vi "Dashboard Main.vi"() -> ()   [LabVIEW 2018]
uses:
  2019_Trobots_5013_Robot/Arm/Arm Positions.ctl
  <vilib>/Utility/miscctls.llb/LVRowAndColumnTypeDef.ctl
  <vilib>/event_ctls.llb/eventvkey.ctl
  <vilib>/Rock Robotics/Network Tables/NT Read Numeric Array.vi
  <vilib>/Rock Robotics/WPI/Dashboard/WPI_DashboardLogging Global.vi
panel:
  in  "Camera Settings Right":T1={"Frame Rate"=30, "Compression"=30, "Size"=1, "DB Camera Config"=FALSE} {"Frame Rate" scale=1.0..30.0; "Compression" scale=100.0..-1.0; "Size" items=["640x480", "320x240", "160x120"]}
  in  "Camera Name Right":string(combo)="No Camera Selection"
  out "Camera Perf":string
  in  "Camera Settings":T1={"Frame Rate"=30, "Compression"=30, "Size"=1, "DB Camera Config"=FALSE} {"Frame Rate" scale=1.0..30.0; "Compression" scale=100.0..-1.0; "Size" items=["640x480", "320x240", "160x120"]}
  in  "TCP":refnum<k5>
  in  "Rec Mode":enum32{"Stop", "Record", "Playback"}(radio)
  out "Robot IP":string
  out "Image Message":string="Timeout in Camera Communications"
  in  "Dashboard Tab":T2(tab)=enum."Custom"
  in  "Select Auto":string(combo)="Select Autonomous ..."
  out "NT Connection":bool
  out "MotorChart R":cluster{"Numeric":dbl, "Numeric":dbl}(graph)
  out "MotorChart L":cluster{"Numeric":dbl, "Numeric":dbl}(graph)
  out "MotorSliders R":cluster{"MotorSlide1":dbl, "MotorSlide2":dbl} {"MotorSlide2" scale=-1.0..1.0 scale format="%#_2e"; "MotorSlide1" scale=-1.0..1.0 scale format="%#_2e"}
  out "MotorSliders L":cluster{"MotorSlide1":dbl, "MotorSlide2":dbl} {"MotorSlide2" scale=-1.0..1.0 scale format="%#_2e"; "MotorSlide1" scale=-1.0..1.0 scale format="%#_2e"}
  out "JS1 Z":dbl(slide) scale=-1.0..1.0 scale format="%#_2e"
  out "JS1 Graph":cluster{"X":dbl, "Y":dbl}[](graph)
  out "JS1 Buttons":T3
  out "JS2 Z":dbl(slide) scale=-1.0..1.0 scale format="%#_2e"
  out "JS2 Graph":cluster{"X":dbl, "Y":dbl}[](graph)
  out "JS2 Buttons":T3
  out "Mode":T4(ring)=enum."Auto Disabled"
  out "Right Camera Perf":cluster{"Bandwidth (Mbps)":dbl, "FPS":dbl}
  out "Camera Image Right":T5(plugin-control)
  in  "DB/String 9":string
  in  "DB/String 8":string
  in  "DB/String 7":string
  in  "DB/String 6":string
  in  "DB/String 5":string
  in  "DB/String 4":string
  in  "DB/String 3":string
  in  "DB/String 2":string
  in  "DB/String 1":string
  in  "DB/String 0":string
  in  "DB/Slider 0":dbl(slide) scale=0.0..5.0
  in  "DB/Slider 1":dbl(slide) scale=0.0..5.0
  in  "DB/Slider 2":dbl(slide) scale=0.0..5.0
  in  "DB/Slider 3":dbl(slide) scale=0.0..5.0
  out "DB/LED 3":bool
  out "DB/LED 2":bool
  out "DB/LED 1":bool
  out "DB/LED 0":bool
  in  "DB/Button 3":bool
  in  "DB/Button 2":bool
  in  "DB/Button 1":bool
  in  "DB/Button 0":bool caption="New Name"
  in  "Array":bool[](array[boolean])
  in  "Set":bool
  in  "Elbow Angle":dbl
  in  "Shoulder Angle":dbl
  in  "Wrist Angle":dbl
  in  "Turret Angle":dbl
  in  "Arm Positions":T6
  out "Elbow":dbl format="%#.1f"
  out "Turret":dbl format="%#.1f"
  out "Shoulder":dbl format="%#.1f"
  out "Wrist":dbl format="%#.1f"
  out "Gyro":dbl(knob) scale=-180.0..180.0
  in  "Test Slider":dbl(slide) scale=0.0..100.0 scale format="%#_3g"
  in  "On/Off":bool caption="Solenoid"
  in  "Test Name":u16(ring) items=["Select the test to run..."]
  in  "Test Tree":string(tree)
  in  "Motor":cluster{"Value":dbl, "Enable":bool} {"Value" scale=-1.0..1.0 scale format="%#_3g"}
  out "Progress":T7 {"Test Progress" scale=0.0..100.0}
  in  "Rev/Fwd":cluster{"Forward":bool, "Reverse":bool}
  in  "Test Ring":u16(ring) items=["Monochrome", "Color"]
  out "Cmd Status":string
  in  "Execute Command":bool
  in  "Command Params":string[][](table)
  in  "Command Selection":i32(listbox)
  in  "CheckList":i32(listbox)
  out "Tree":string(tree)
  out "Camera Image":T5(plugin-control)
  out "Background":bool
  in  "Camera Name":string(combo)="No Camera Selection"
  # "HW"
  # "HW"
  # "Joysticks"
  # "Drive Motors"
  # "Front"
  # "Right"
  # "Left"
  # "Back"
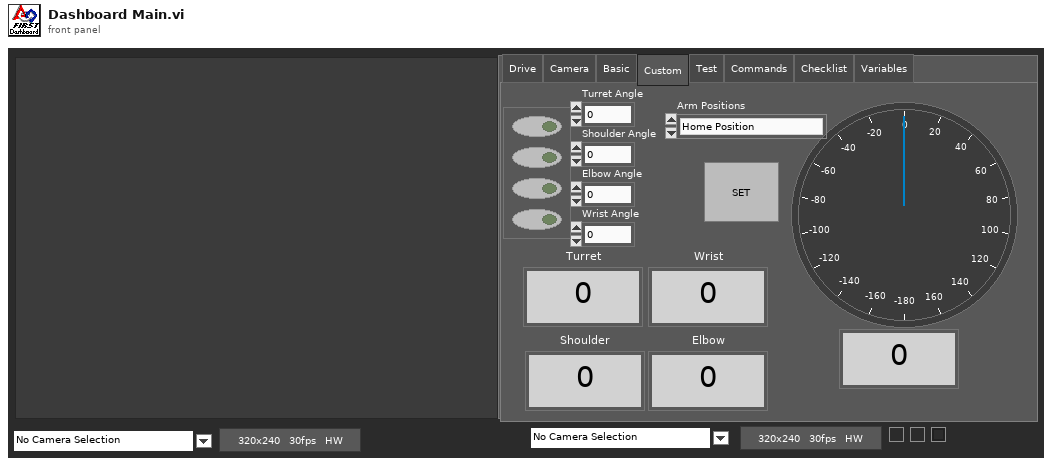
[diagram p1: front panel]
types:
  T1 = cluster{"Frame Rate":i32, "Compression":i32, "Size":u16, "DB Camera Config":bool}
  T2 = enum32{"Drive", "Camera", "Basic", "Custom", "Test", "Commands", "Checklist", "Variables"}
  T3 = cluster{bool, bool, bool, bool, bool, bool, bool, bool, bool, bool, bool, bool}
  T4 = enum8{"Tele-Op Disabled", "Tele-Op Enabled", "Auto Disabled", "Auto Enabled", "Test Disabled", "Test Enabled", "Disconnected", "No Code", "E-Stop"}
  T5 = typedef "IMAQ Image.ctl" = refnum<image>
  T6 = typedef "Arm Positions.ctl" = enum16{"Home Position", "Safe Position", "Hatch - Ground", "Hatch - Low", "Hatch - Middle", "Hatch - High", "Hatch - High 2", "Cargo - Low", "Cargo - Middle", "Cargo - High", "Cargo - Loading Station", "Hatch - Loading Station", "Cargo - Ground", "Turret - Left", "Turret - Front", "Turret - Right", "Turret - Back", "Climbing - Forward", "Hatch - Middle2"}
  T7 = cluster{"Test Progress":u8, "Test Progress Text":string}
  T8 = cluster{"Save Path":path, "Interval (s)":dbl, "Keep":i32}
  T9 = typedef "Image Type" = u32
  T10 = cluster{"IDs":cluster{"RPC field ID":u16, "Unique ID":u16}, "String":string}
  T11 = cluster{"Error Strings":string, "Disable Counts":cluster{u16, u16}, "Rail Faults":cluster{u16, u16, u16}, "Robot IP":string, "DB Mode":u8, "Event Info":cluster{"Name":string, "Type":u8, "Number":u16, "Replay":u8}}
  T12 = cluster{"Storage":cluster{"Disk Free":u64, "RAM Block":u32, "RAM free":u32}, "CPU Utilization":cluster{"CPU % ISR":sgl, "CPU % Time Crit":sgl, "CPU % Timed Str":sgl, "CPU % High":sgl, "CPU % Above":sgl, "CPU % Normal":sgl, "CPU % Low":sgl}, "CAN":cluster{"% Bus Utilization":sgl, "Bus Off Cnt":u32, "TX_FIFO Full Cnt":u32, "Receive Error Cnt":u8, "Transmit Error Cnt":u8}, "HID":cluster{"HID Outputs":u32, "Rumble Low":u16, "Rumble High":u16}[]}
  T13 = cluster{"Status bits":cluster{"Test Mode":bool, "Autonomous":bool, "Enabled":bool, "Code Start":bool, "Brownout":bool, "Reserved 2":bool, "Reserved 3":bool, "E-Stop":bool}, "Code Trace":cluster{"Disabled":bool, "TeleOp":bool, "Auto":bool, "Test":bool}, "Controller Type":enum16{"unknown", "cRIO", "roboRio"}, "Code?":enum16{"unknown", "noCode", "code"}, "Battery V":dbl}
  T14 = cluster{"Control Bits":cluster{"TestMode":bool, "Autonomous":bool, "Enabled":bool, "FMS Present":bool, bool, bool, bool, "E-Stop":bool}, "Team Station ":u8, "Countdown":sgl, "Joystick Values":cluster{"Axes":dbl[], "Buttons":bool[], "POVs":i16[]}[]}
  T15 = cluster{"Axes":dbl[], "Buttons":bool[], "POVs":i16[]}[]
  T16 = cluster{"Axes":dbl[], "Buttons":bool[], "POVs":i16[]}
  T17 = cluster{"Buttons[0]":bool, "Buttons[1]":bool, "Buttons[2]":bool, "Buttons[3]":bool, "Buttons[4]":bool, "Buttons[5]":bool, "Buttons[6]":bool, "Buttons[7]":bool, "Buttons[8]":bool, "Buttons[9]":bool, "Buttons[10]":bool, "Buttons[11]":bool}
  T18 = cluster{"Camera Image":refnum<vi>, "Dashboard Tab":refnum<vi>, "Background":refnum<vi>, "Rec Mode":refnum<vi>, "Test Slider":refnum<vi>, "On/Off ":refnum<vi>, "Test Ring":refnum<vi>, "Rev/Fwd":refnum<vi>, "Test Name":refnum<vi>, "Motor":refnum<vi>, "Progress":refnum<vi>, "CheckList":refnum<vi>, "Tree":refnum<vi>, "Test Tree":refnum<vi>, "Command Params":refnum<vi>, "Command Selection":refnum<vi>, "Execute Command":refnum<vi>, "Cmd Status":refnum<vi>, "Camera Settings":refnum<vi>, "Camera Name":refnum<vi>, "Camera Perf":refnum<vi>, "Camera Settings Right":refnum<vi>, "Camera Name Right":refnum<vi>, "Camera Image Right":refnum<vi>}
  T19 = cluster{"Global Rectangle":i32[], "Contours":cluster{"Contour Type":u32, "ROI Type":u32, "Points":i32[]}[]}
  T20 = cluster{"Camera Name":string, string, "Saved DB Images Info":cluster{"Save Path":path, "Interval (s)":dbl, "Keep":i32}}
  T21 = cluster{"Camera Name Right":string, string, "Saved DB Images Info":cluster{"Save Path":path, "Interval (s)":dbl, "Keep":i32}}
  T22 = cluster{"Operation":enum16{"Update", "Clear"}, "Color Box":u32}[]
  T23 = typedef "eventvkey.ctl" = enum16{"ASCII", "Enter", "Return", "Shift", "Ctrl", "Alt", "Cmd", "Opt", "Caps", "NumLock", "Clear", "Break", "Up", "Down", "Left", "Right", "Insert", "Delete", "Home", "End", "PageUp", "PageDown", "Escape", "Help", "Pause", "ScrollLock", "F1", "F2", "F3", "F4", "F5", "F6", "F7", "F8", "F9", "F10", "F11", "F12", "F13", "F14", "F15", "F16", "F17", "F18", "F19", "F20", "F21", "F22", "F23", "F24", "Play", "VolumeUp", "VolumeDown", "Mute", "Two Byte Char"}
  T24 = cluster{"Image Size":bool, "Image Type":bool, "Pixel Value":bool, "ROI Information":bool, "Zoom Factor":bool}
  T25 = cluster{"Operation":enum16{"Update", "Clear"}, "Color Box":u32}
  T26 = typedef "LVRowAndColumnTypeDef.ctl" = cluster{"Row":i32, "Column":i32}
  T27 = cluster{"Shift":bool, "Ctrl":bool, "Alt":bool, "Cmd":bool, "Opt":bool}
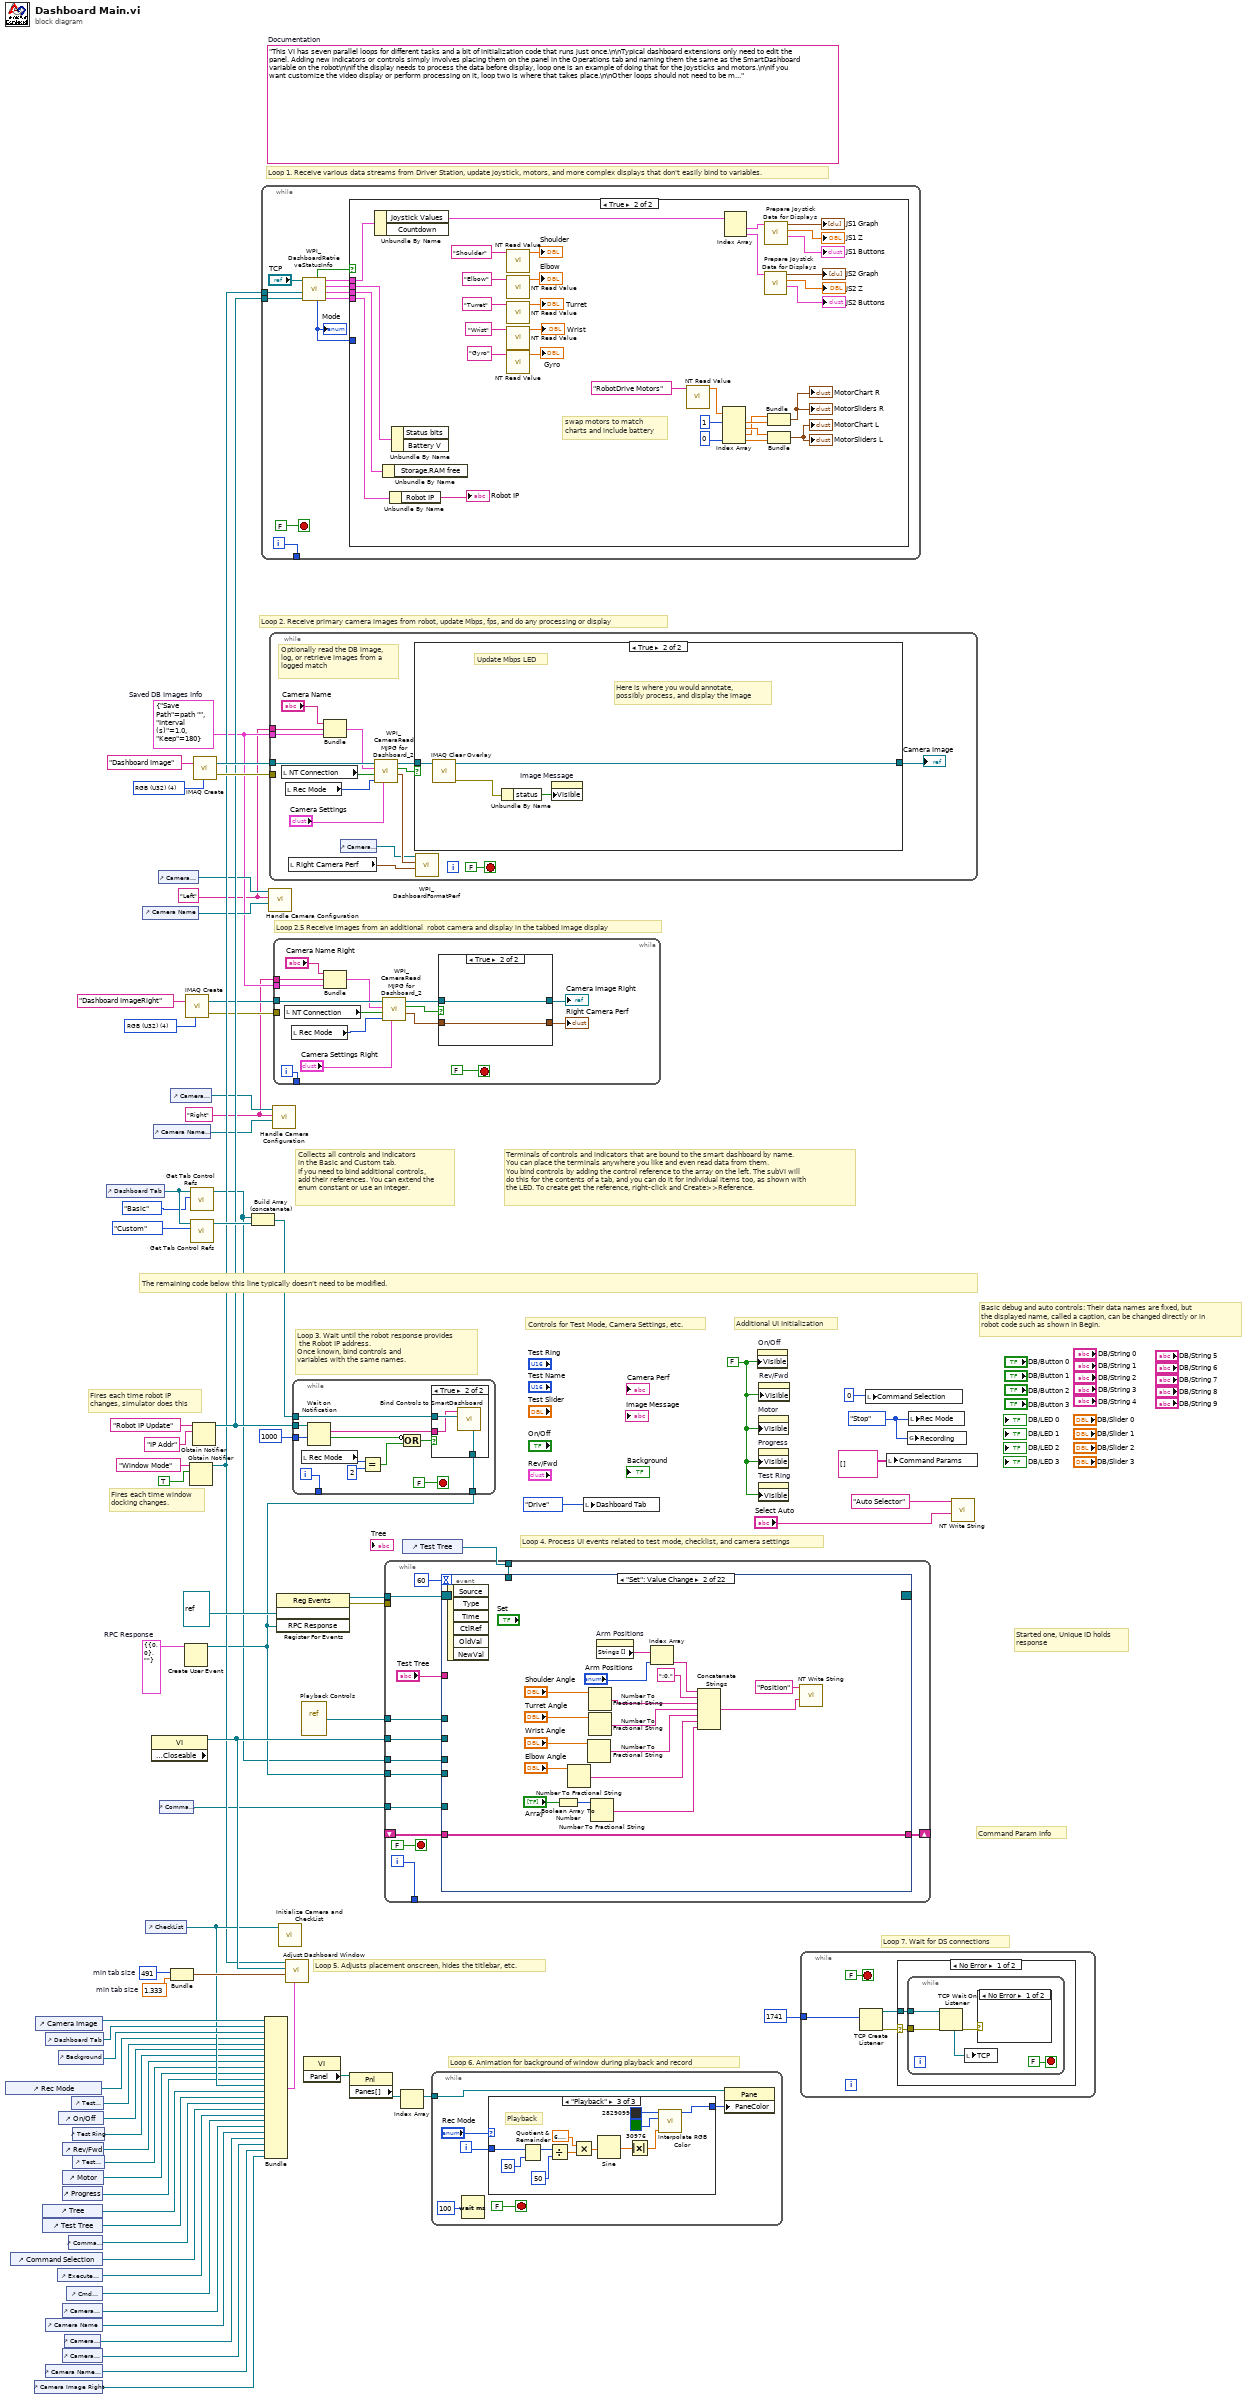
[diagram p0: block diagram]
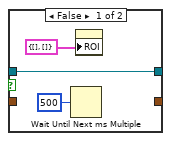
[diagram p2: hidden frame]
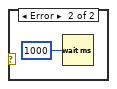
[diagram p3: hidden frame]
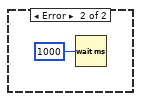
[diagram p4: hidden frame]
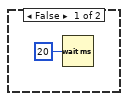
[diagram p5: hidden frame]
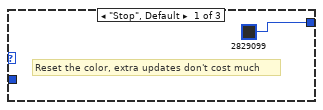
[diagram p6: hidden frame]
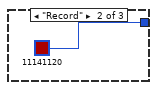
[diagram p7: hidden frame]
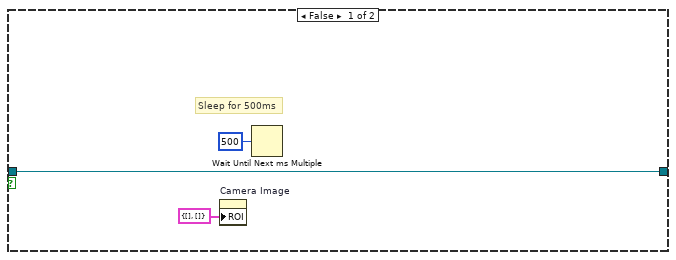
[diagram p9: hidden frame]
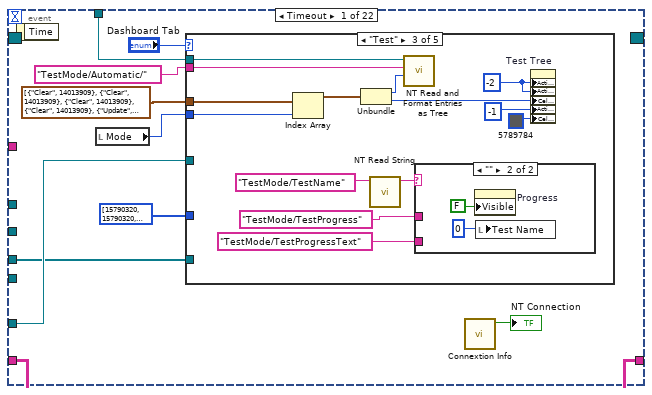
[diagram p10: hidden frame]
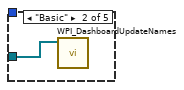
[diagram p12: hidden frame]
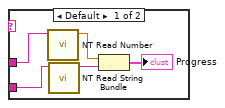
[diagram p13: hidden frame]
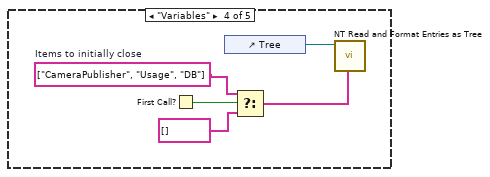
[diagram p14: hidden frame]
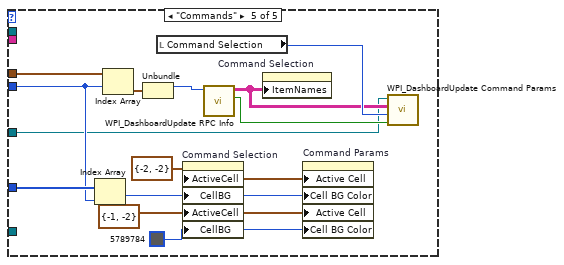
[diagram p15: hidden frame]
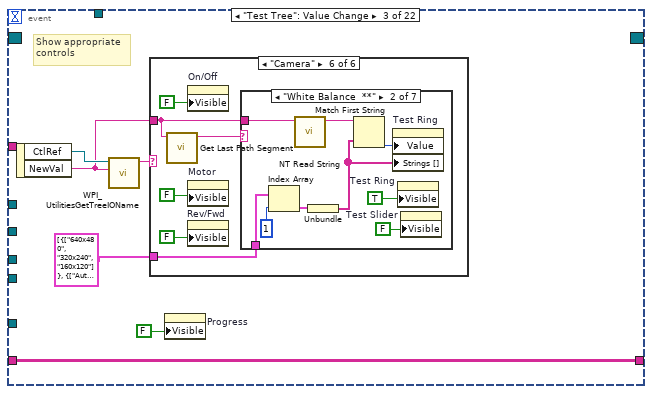
[diagram p16: hidden frame]
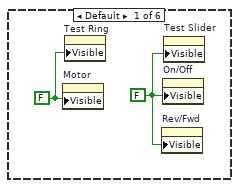
[diagram p17: hidden frame]
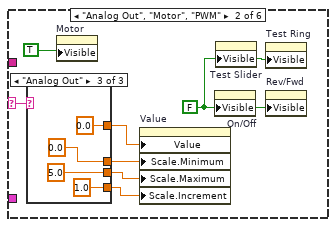
[diagram p18: hidden frame]
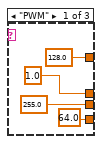
[diagram p19: hidden frame]
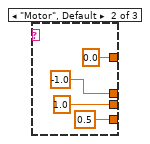
[diagram p20: hidden frame]
diagram:
  w3 = T8 {"Save Path"=path "", "Interval (s)"=1.0, "Keep"=180}  # Saved DB Images Info
  w2 = "Right"
  w1 = "Left"
  w13 = T9 4 items=["Grayscale (U8)", "Grayscale (I16)", "Grayscale (SGL)", "Complex (CSG)", "RGB (U32)", "HSL (U32)", "RGB (U64)"] ("Image Type")
  w29 = T10 {"IDs"={"RPC field ID"=0, "Unique ID"=0}, "String"=""}  # RPC Response
  w52 = 491  # min tab size
  w51 = 1.333  # min tab size
  w59 = enum32{"Stop", "Record", "Playback"}."Stop" ("Rec Mode")
  w36 = FALSE ("Visible")
  (unwired) "This VI has seven parallel loops for different tasks and a bit of initialization code that runs just once.\n\nTypical dashboard extensions only need to edit the panel. Adding new indicators or controls simply involves placing them on the panel in the Operations tab and naming them the same as the SmartDashboard variable on the robot\n\nIf the display needs to process the data before display, loop one is an example of doing that for the joysticks and motors.\n\nIf you want customize the video display or perform processing on it, loop two is where that takes place.\n\nOther loops should not need to be modified. They are pretty standard, and document the task they perform."  # Documentation
  w76 = T9 4 items=["Grayscale (U8)", "Grayscale (I16)", "Grayscale (SGL)", "Complex (CSG)", "RGB (U32)", "HSL (U32)", "RGB (U64)"] ("Image Type")
  # "Loop 2.5 Receive images from an additional  robot camera and display in the tabbed image display"
  # "Command Param Info"
  # "Started one, Unique ID holds\nresponse"
  # "Loop 7. Wait for DS connections"
  # "Basic debug and auto controls: Their data names are fixed, but\nthe displayed name, called a caption, can be changed directly or in\nrobot code such as shown in Begin."
  # "Controls for Test Mode, Camera Settings, etc."
  # "Additional UI Initialization"
  # "Loop 6. Animation for background of window during playback and record"
  # "Fires each time robot IP\nchanges, simulator does this"
  # "Fires each time window\ndocking changes."
  # "Collects all controls and indicators\nin the Basic and Custom tab.\nIf you need to bind additional controls,\nadd their references. You can extend the\nenum constant or use an integer."
  # "The remaining code below this line typically doesn't need to be modified."
  # "Loop 4. Process UI events related to test mode, checklist, and camera settings"
  # "Terminals of controls and indicators that are bound to the smart dashboard by name.\nYou can place the terminals anywhere you like and even read data from them.\nYou bind controls by adding the control reference to the array on the left. The subVI will\ndo this for the contents of a tab, and you can do it for individual items too, as shown with\nthe LED. To create get the reference, right-click and Create>>Reference."
  # "Loop 3. Wait until the robot response provides\n the Robot IP address.\nOnce known, bind controls and\nvariables with the same names."
  # "Loop 5. Adjusts placement onscreen, hides the titlebar, etc."
  # "Loop 1. Receive various data streams from Driver Station, update joystick, motors, and more complex displays that don't easily bind to variables."
  # "Loop 2. Receive primary camera images from robot, update Mbps, fps, and do any processing or display"
  n1 = control-ref of="Rec Mode"() -> (w42:refnum<vi>)
  n2 = control-ref of="Command Selection"() -> (w28:refnum<vi>)
  n3 = control-ref of="Camera Image Right"() -> (w6:refnum<vi>)
  n4 = control-ref of="Camera Image"() -> (w54:refnum<vi>)
  n5 = control-ref of="Tree"() -> (w46:refnum<vi>)
  n6 = control-ref of="Test Tree"() -> (w45:refnum<vi>)
  n7 = control-ref of="Dashboard Tab"() -> (w53:refnum<vi>)
  n8 = control-ref of="Camera Name"() -> (w19:refnum<vi>)
  n9 = control-ref of="Camera Name Right"() -> (w7:refnum<vi>)
  n10 = control-ref of="Execute Command"() -> (w30:refnum<vi>)
  n11 = control-ref of="Background"() -> (w49:refnum<vi>)
  n12 = control-ref of="On/Off"() -> (w40:refnum<vi>)
  n13 = control-ref of="Progress"() -> (w37:refnum<vi>)
  n14 = control-ref of="Camera Settings"() -> (w20:refnum<vi>)
  n15 = control-ref of="Camera Settings Right"() -> (w8:refnum<vi>)
  n16 = control-ref of="Rev/Fwd"() -> (w38:refnum<vi>)
  n17 = control-ref of="Motor"() -> (w43:refnum<vi>)
  n18 = control-ref of="Camera Perf"() -> (w18:refnum<vi>)
  n19 = control-ref of="Cmd Status"() -> (w24:refnum<vi>)
  n20 = control-ref of="Command Params"() -> (w31:refnum<vi>)
  n21 = control-ref of="Test Slider"() -> (w41:refnum<vi>)
  n22 = control-ref of="Test Ring"() -> (w39:refnum<vi>)
  n23 = control-ref of="Test Name"() -> (w44:refnum<vi>)
  n24 = control-ref of="Dashboard Tab"() -> (w57:refnum<vi>)
  n25 = control-ref of="Camera Name"() -> (w21:refnum<vi>)
  n26 = control-ref of="CheckList"() -> (w47:refnum<vi>)
  n27 = property class="VI" props=["Front Panel.Closeable"]() -> (reference out=w58:refnum<vi>)  [unwired: 2 in, 2 out]
  n28 = control-ref of="Camera Name Right"() -> (w9:refnum<vi>)
  n29 = control-ref of="Camera Settings"() -> (w22:refnum<vi>)
  n30 = control-ref of="Command Params"() -> (w23:refnum<vi>)
  n31 = control-ref of="Camera Settings Right"() -> (w10:refnum<vi>)
  n32 = Bundle("min tab size"=w52, "min tab size"=w51) -> (w50:cluster{"min tab size":i32, "min tab size":dbl})  [unwired: 1 in]
  n33 = Create User Event(user event datatype=w29) -> (user event=w25:refnum<user-event>)  [unwired: 1 in, 1 out]
  n34 = call "IMAQ Create"("Image Name"="Dashboard ImageRight", "Image Type"=w13) -> ("New Image"=w12:T5, "error out"=w11:errorcluster)  [unwired: 2 in, 1 out]
  n35 = Obtain Notifier(name (unnamed)="Window Mode", notification data type=TRUE) -> (notifier out=w34:refnum<notifier>)  [unwired: 2 in, 2 out]
  n36 = call <vilib>:"Get Tab Control Refs.vi"("Page Index"=T2."Basic" ("Dashboard Tab"), "TabControl in"=w57) -> ("ControlsOnPage"=w17:refnum<vi>[])  [unwired: 9 in]
  n37 = call <vilib>:"Get Tab Control Refs.vi"("Page Index"=T2."Custom" ("Dashboard Tab"), "TabControl in"=w57) -> ("ControlsOnPage"=w56:refnum<vi>[])  [unwired: 9 in]
  n38 = Obtain Notifier(name (unnamed)="Robot IP Update", notification data type="IP Addr" ("name (unnamed)")) -> (notifier out=w35:refnum<notifier>)  [unwired: 2 in, 2 out]
  n39 = call "IMAQ Create"("Image Name"="Dashboard Image", "Image Type"=w76) -> ("New Image"=w74:T5, "error out"=w73:errorcluster)  [unwired: 2 in, 1 out]
  n40 = Build Array (concatenate)(w17, w56) -> (w55:refnum<vi>[])
  n41 = while {
    tunnel: [w86] -> _
    tunnel: w35 -> [w80]
    tunnel: w34 -> [w77]
    i -> [w86]
    stop <- FALSE stop-if-true
    n42 = call <vilib>:"WPI_DashboardRetrieveStatusInfo.vi"("Binding Refnum"=w80, "Window Mode Notifier"=w77, "TCP Cnx"="TCP") -> ("Power and Errors"=w81:T11, "Robot Metrics"=w84:T12, "Status Info"=w85:T13, "Control Info"=w82:T14, "Robot Mode"=w79:T4, "Process?"=w83:bool)  [unwired: 3 in]
    "Mode" <- w79
    n43 = case shown="True" w83 {
      tunnel: w85 -> [_ w122]
      tunnel: w84 -> [_ w121]
      tunnel: w82 -> [_ w120]
      tunnel: w81 -> [_ w119]
      tunnel: w79 -> [_ _]
      frame False {
        n44 = Wait (ms)(milliseconds to wait=u32 20) -> ()  [unwired: 1 out]
      }
      frame True {
        # "swap motors to match\ncharts and include battery"
        n45 = Unbundle By Name(w120) -> ("Joystick Values"=w110:T15)  [unwired: 1 out]
        n46 = Unbundle By Name(w121) -> ()  [unwired: 1 out]
        n47 = Unbundle By Name(w119) -> ("Robot IP"=→"Robot IP":string)
        n48 = Unbundle By Name(w122) -> ()  [unwired: 2 out]
        n49 = call-poly <vilib>:"NT Read Value.vi"("Name"="Shoulder") -> ("Numeric"=→"Shoulder":dbl)  [unwired: 9 in, 1 out]
        n50 = call-poly <vilib>:"NT Read Value.vi"("Name"="Elbow") -> ("Numeric"=→"Elbow":dbl)  [unwired: 9 in, 1 out]
        n51 = call-poly <vilib>:"NT Read Value.vi"("Name"="Turret") -> ("Numeric"=→"Turret":dbl)  [unwired: 9 in, 1 out]
        n52 = call-poly <vilib>:"NT Read Value.vi"("Name"="Wrist") -> ("Numeric"=→"Wrist":dbl)  [unwired: 9 in, 1 out]
        n53 = call-poly <vilib>:"NT Read Value.vi"("Name"="Gyro") -> ("Numeric"=→"Gyro":dbl)  [unwired: 9 in, 1 out]
        n54 = call-poly <vilib>:"NT Read Value.vi"("Name"="RobotDrive Motors") -> ("Numeric Array"=w100:dbl[])  [unwired: 9 in, 1 out]
        n55 = Index Array(array=w100, index #1=1, index #4=0) -> (element #1=w114:dbl, element #2=w115:dbl, element #3=w113:dbl, element #4=w118:dbl)  [unwired: 2 in]
        n56 = Index Array(array=w110) -> (element #1=w109:T16, element #2=w105:T16)  [unwired: 2 in]
        n57 = call "Prepare Joystick Data for Displays.vi"("Joystick Values"=w105) -> ("Buttons"=→"JS2 Buttons":T17, "Z Axis"=→"JS2 Z":dbl, "Cartesian Data"=→"JS2 Graph":cluster{"X axis":dbl, "X axis":dbl}[])  [unwired: 8 in]
        n58 = call "Prepare Joystick Data for Displays.vi"("Joystick Values"=w109) -> ("Buttons"=→"JS1 Buttons":T17, "Z Axis"=→"JS1 Z":dbl, "Cartesian Data"=→"JS1 Graph":cluster{"X axis":dbl, "X axis":dbl}[])  [unwired: 8 in]
        n59 = Bundle("Numeric"=w113, "Numeric"=w114) -> (→"MotorChart R" →"MotorSliders R":cluster{"Numeric":dbl, "Numeric":dbl})  [unwired: 1 in]
        n60 = Bundle("Numeric"=w115, "Numeric"=w118) -> (→"MotorChart L" →"MotorSliders L":cluster{"Numeric":dbl, "Numeric":dbl})  [unwired: 1 in]
      }
    }
  }
  n61 = Bundle("Camera Image"=w54, "Dashboard Tab"=w53, "Background"=w49, "Rec Mode"=w42, "Test Slider"=w41, "On/Off"=w40, "Test Ring"=w39, "Rev/Fwd"=w38, "Test Name"=w44, "Motor"=w43, "Progress"=w37, "CheckList"=w47, "Tree"=w46, "Test Tree"=w45, "Command Params"=w31, "Command Selection"=w28, "Execute Command"=w30, "Cmd Status"=w24, "Camera Settings"=w20, "Camera Name"=w19, "Camera Perf"=w18, "Camera Settings Right"=w8, "Camera Name Right"=w7, "Camera Image Right"=w6) -> (w48:T18)  [unwired: 1 in]
  n62 = call "Handle Camera Configuration.vi"("CameraNameRef"=w21, "Display Name"=w1, "ClusterRef"=w22) -> ()  [unwired: 9 in]
  n63 = while {
    tunnel: w74 -> [w136]
    tunnel: w73 -> [_]
    tunnel: w3 -> [w129]
    tunnel: w1 -> [w126]
    stop <- FALSE stop-if-true
    # "Optionally read the DB image,\nlog, or retrieve images from a\nlogged match"
    n64 = local read "NT Connection"() -> (w130:bool)
    n65 = local read "Rec Mode"() -> (w133:enum32{"Stop", "Record", "Playback"})
    n66 = local read "Right Camera Perf"() -> (w124:cluster{"Bandwidth (Mbps)":dbl, "FPS":dbl})
    n67 = Bundle("Camera Name"="Camera Name", w126, "Saved DB Images Info"=w129) -> (w128:T20)  [unwired: 1 in]
    n68 = control-ref of="Camera Perf"() -> (w123:refnum<vi>)
    n69 = call <vilib>:"WPI_CameraRead MJPG for Dashboard_2.vi"("Camera Settings"="Camera Settings", "Rec Mode"=w133, "NT Connection"=w130, "Capture Info"=w128, "Image in"=w136) -> ("perf info"=w125:cluster{"Bandwidth (Mbps)":dbl, "fps":dbl}, "Active"=w134:bool, "Image\\ out"=w135:T5)  [unwired: 4 in]
    n70 = case shown="True" w134 {
      tunnel: w135 -> [w139 w142]
      tunnel: [w139 w141] -> w131
      frame False {
        # "Sleep for 500ms"
        n71 = property on="Camera Image" class="ImageControl"("ROI"=T19 {"Global Rectangle"=[], "Contours"=[]}) -> ()  [unwired: 2 in, 2 out]
        n72 = Wait Until Next ms Multiple(millisecond multiple=u32 500) -> ()  [unwired: 1 out]
      }
      frame True {
        # "Here is where you would annotate,\npossibly process, and display the image"
        # "Update Mbps LED"
        n73 = call "IMAQ Clear Overlay"("Image"=w142) -> ("error out"=w143:errorcluster, "Image Out"=w141:T5)  [unwired: 2 in, 7 out]
        n74 = Unbundle By Name(w143) -> ("status"=w144:bool)
        n75 = property on="Image Message" class="Str"("Visible"=w144) -> ()  [unwired: 2 in, 2 out]
      }
    }
    "Camera Image" <- w131
    n76 = call <vilib>:"WPI_DashboardFormatPerf.vi"("Right Camera Perf"=w124, "Performance"=w125, "String in"=w123) -> ()  [unwired: 9 in]
  }
  n77 = call "Handle Camera Configuration.vi"("CameraNameRef"=w9, "Display Name"=w2, "ClusterRef"=w10) -> ()  [unwired: 9 in]
  n78 = while {
    tunnel: w12 -> [w159]
    tunnel: w11 -> [_]
    tunnel: [w154] -> _
    tunnel: w3 -> [w150]
    tunnel: w2 -> [w147]
    i -> [w154]
    stop <- FALSE stop-if-true
    n79 = local read "NT Connection"() -> (w151:bool)
    n80 = local read "Rec Mode"() -> (w158:enum32{"Stop", "Record", "Playback"})
    n81 = Bundle("Camera Name Right"="Camera Name Right", w147, "Saved DB Images Info"=w150) -> (w149:T21)  [unwired: 1 in]
    n82 = call <vilib>:"WPI_CameraRead MJPG for Dashboard_2.vi"("Camera Settings"="Camera Settings Right", "Rec Mode"=w158, "NT Connection"=w151, "Capture Info"=w149, "Image in"=w159) -> ("perf info"=w145:cluster{"Bandwidth (Mbps)":dbl, "fps":dbl}, "Active"=w153:bool, "Image\\ out"=w156:T5)  [unwired: 4 in]
    n83 = case shown="True" w153 {
      tunnel: w156 -> [w161 w164]
      tunnel: [w161 w164] -> w152
      tunnel: [_ w163] -> w146
      tunnel: w145 -> [_ w163]
      frame False {
        n84 = Wait Until Next ms Multiple(millisecond multiple=u32 500) -> ()  [unwired: 1 out]
        n85 = property on="Camera Image Right" class="ImageControl"("ROI"=T19 {"Global Rectangle"=[], "Contours"=[]}) -> ()  [unwired: 2 in, 2 out]
      }
      frame True {
      }
    }
    "Camera Image Right" <- w152
    "Right Camera Perf" <- w146
  }
  n86 = register-events(refnum<vi> refnum, w25) -> (reference out=w63:refnum<event-registration>, error out=w62:errorcluster)  [unwired: 2 in]
  n87 = call "Initialize Camera and CheckList.vi"("ListBox in"=w47) -> ()  [unwired: 11 in]
  n88 = call "Adjust Dashboard Window.vi"("Sizing Refnums"=w48, "Size Constraints"=w50, "VI"=w58, "WIn Mode"=w34) -> ()  [unwired: 8 in]
  n89 = while {
    tunnel: w55 -> [w176]
    tunnel: w35 -> [w174]
    tunnel: [w172] -> _
    tunnel: u32 1000 ("milliseconds to wait") -> [w171]
    tunnel: w25 -> [w165]
    i -> [w172]
    stop <- FALSE stop-if-true
    n90 = local read "Rec Mode"() -> (w167:enum32{"Stop", "Record", "Playback"})
    n91 = Wait on Notification(notifier=w174, timeout in ms (-1)=w171) -> (notification=w173:string, timed out?=w169:bool)  [unwired: 2 in, 2 out]
    n92 = Equal?(x=w167, y=u16 2 ("Rec Mode")) -> (x = y?=w168:bool)
    n93 = Compound Arithmetic op=OR(invert w169, w168) -> (w170:bool)
    n94 = case shown="True" w170 {
      tunnel: w176 -> [_ w179]
      tunnel: w173 -> [_ w178]
      tunnel: w165 -> [_ w177]
      frame False {
      }
      frame True {
        n95 = call <vilib>:"Bind Controls to SmartDashboard.vi"("RPC ref"=w177, "Bound Control Refs"=w179, "Server IP Address"=w178) -> ()  [unwired: 9 in]
      }
    }
  }
  n96 = vi-ref "Playback Controls.vi"() -> (w64:refnum<vi>)
  n97 = property class="VI"() -> ("Panel"=w66:refnum<vi>)  [unwired: 2 in, 2 out]
  n98 = property class="Pnl"(reference=w66) -> ("Panes[]"=w67:refnum<vi>[])  [unwired: 1 in, 2 out]
  n99 = Index Array(array=w67) -> (element=w65:refnum<vi>)  [unwired: 1 in]
  n100 = control-ref of="Test Tree"() -> (w68:refnum<vi>)
  n101 = while {
    tunnel: [w189] -> _
    tunnel: w68 -> [w188]
    tunnel: w64 -> [w187]
    tunnel: w63 -> [w186]
    tunnel: w62 -> [_]
    tunnel: w58 -> [w185]
    tunnel: w25 -> [w184]
    tunnel: w23 -> [w183]
    shift-right: [w182] -> _
    shift-left: _ -> [w181]
    tunnel: w17 -> [w180]
    i -> [w189]
    stop <- FALSE stop-if-true
    n102 = event shown="[1] \"Set\": Value Change" {
      selector: w186 -> [_ _ _ _ _ _ _ _ _ _ _ _ _ _ _ _ _ _ _ _ _ _]
      dyn-events: [_ _ _ _ _ _ _ _ _ _ _ _ _ _ _ _ _ w467 _ _ _ _] -> _
      timeout: u32 60 ("milliseconds to wait") -> [_ _ _ _ _ _ _ _ _ _ _ _ _ _ _ _ _ _ _ _ _ _]
      tunnel: w188 -> [w201 _ _ _ _ _ _ _ _ _ _ _ _ _ _ _ _ _ _ _ _ _]
      tunnel: "Test Tree" -> [_ _ _ _ _ _ _ _ _ _ _ _ w434 w442 w444 w448 w456 _ _ _ _ _]
      tunnel: w187 -> [_ _ _ _ _ _ _ _ _ _ _ _ _ _ _ _ _ w469 _ w487 _ _]
      tunnel: w185 -> [_ _ _ _ _ _ _ _ _ _ _ _ _ _ _ _ _ w465 _ _ _ _]
      tunnel: w184 -> [_ _ _ _ _ _ _ _ _ _ _ _ _ _ _ _ _ w463 _ _ _ _]
      tunnel: w183 -> [w196 _ _ _ _ _ _ w385 _ _ _ _ _ _ _ _ _ _ _ _ _ _]
      tunnel: [w195 w260 w262 w364 w369 w378 w382 w383 w392 w402 w409 w421 w433 w440 w443 w447 w455 w462 w482 w484 w488 w501] -> w182
      tunnel: w181 -> [w195 w260 w262 w364 w369 w378 w382 w383 _ _ w409 w421 w433 w440 w443 w447 w455 w462 w482 w484 w488 w501]
      tunnel: w180 -> [w193 _ _ _ _ _ _ _ _ _ _ _ _ _ _ _ _ _ _ _ _ _]
      event Timeout {
        n103 = event-data() -> ()  [unwired: 1 in, 1 out]
        n104 = local read "Mode"() -> (w198:T4)
        n105 = case shown="\"Test\"" "Dashboard Tab" {
          tunnel: w201 -> [_ _ w217 _ _]
          tunnel: "TestMode/Automatic/" ("Name Pattern") -> [_ _ w216 _ _]
          tunnel: T22 [{"Operation"=enum."Clear", "Color Box"=14013909}, {"Operation"=enum."Clear", "Color Box"=14013909}, {"Operation"=enum."Clear", "Color Box"=14013909}, {"Operation"=enum."Clear", "Color Box"=14013909}, {"Operation"=enum."Update", "Color Box"=14013909}, {"Operation"=enum."Update", "Color Box"=16777215}, {"Operation"=enum."Clear", "Color Box"=14013909}, {"Operation"=enum."Clear", "Color Box"=14013909}, {"Operation"=enum."Clear", "Color Box"=14013909}] -> [_ _ w209 _ w237]
          tunnel: w198 -> [_ _ w208 _ w236]
          tunnel: u32[] [15790320, 15790320, 15790320, 15790320, 16777215, 16777215, 15790320, 15790320, 15790320] -> [_ _ _ _ w242]
          tunnel: w196 -> [_ _ _ _ w230]
          tunnel: w193 -> [_ w203 _ _ _]
          frame "Custom", Default {
          }
          frame "Basic" {
            n106 = call <vilib>:"WPI_DashboardUpdateNames.vi"("Controls on Tab"=w203) -> ()  [unwired: 11 in]
          }
          frame "Test" {
            w215 = -2 ("Active Item:Row Number")
            n107 = Index Array(array=w209, index=w208) -> (element=w210:T25)
            n108 = Unbundle(w210) -> ("Operation"=w211:enum16{"Update", "Clear"}, "Color Box"=w212:u32)
            n109 = call <vilib>:"NT Read String.vi"("Name"="TestMode/TestName") -> ("String"=w206:string)  [unwired: 9 in, 1 out]
            n110 = call <vilib>:"NT Read and Format Entries as Tree.vi"("Operation"=w211, "Name Pattern"=w216, "Tree Refnum"=w217) -> ()  [unwired: 7 in, 2 out]
            n111 = case shown="\"\"" w206 {
              tunnel: "TestMode/TestProgress" ("Name") -> [w219 _]
              tunnel: "TestMode/TestProgressText" ("Name") -> [w218 _]
              frame Default {
                n112 = call <vilib>:"NT Read Number.vi"("Name"=w219) -> ("Numeric"=w220:dbl)  [unwired: 9 in, 1 out]
                n113 = call <vilib>:"NT Read String.vi"("Name"=w218) -> ("String"=w221:string)  [unwired: 9 in, 1 out]
                n114 = Bundle("Numeric"=w220, "String"=w221) -> (→"Progress":cluster{"Numeric":dbl, "String":string})  [unwired: 1 in]
              }
              frame "" {
                n115 = property on="Progress" class="Clust (strict)"("Visible"=FALSE) -> ()  [unwired: 2 in, 2 out]
                n116 = local write "Test Name"(u16 0) -> ()
              }
            }
            n117 = property on="Test Tree" class="Tree (strict)"("Active Item Row Number"=w215, "ActiveColNum"=w215, "CellBG"=w212, "Active Item Row Number"=-1 ("Active Item:Row Number"), "CellBG"=u32 5789784 ("Color Box")) -> ()  [unwired: 2 in, 2 out]
          }
          frame "Variables" {
            w227 = string[] ["CameraPublisher", "Usage", "DB"]  # Items to initially close
            n118 = First Call?() -> (First Call?: T/F=w228:bool)
            n119 = control-ref of="Tree"() -> (w229:refnum<vi>)
            n120 = Select(t=w227, s=w228, f=string[] []) -> (s? t:f=w225:string[])
            n121 = call <vilib>:"NT Read and Format Entries as Tree.vi"("Tags to  Close"=w225, "Tree Refnum"=w229) -> ()  [unwired: 8 in, 2 out]
          }
          frame "Commands" {
            w238 = u32 5789784 ("Color Box")
            w239 = T26 {"Row"=-1, "Column"=-2} ("Active Cell:Active Cell")
            w241 = T26 {"Row"=-2, "Column"=-2} ("Active Cell:Active Cell")
            n122 = Index Array(array=w242, index=w236) -> (element=w240:u32)
            n123 = Index Array(array=w237, index=w236) -> (element=w235:T25)
            n124 = Unbundle(w235) -> ("Operation"=w234:enum16{"Update", "Clear"})  [unwired: 1 out]
            n125 = local read "Command Selection"() -> (w233:i32)
            n126 = property on="Command Selection" class="MCListbox (strict)"("ActiveCell"=w241, "CellBG"=w240, "ActiveCell"=w239, "CellBG"=w238) -> ()  [unwired: 2 in, 2 out]
            n127 = call <vilib>:"WPI_DashboardUpdate RPC Info.vi"("Operation"=w234) -> ("update"=w232:bool, "commands"=w231:string[][])  [unwired: 9 in]
            n128 = property on="Command Selection" class="MCListbox (strict)"("ItemNames"=w231) -> ()  [unwired: 2 in, 2 out]
            n129 = property on="Command Params" class="Tbl (strict)"("Active Cell"=w241, "Cell BG Color"=w240, "Active Cell"=w239, "Cell BG Color"=w238) -> ()  [unwired: 2 in, 2 out]
            n130 = call <vilib>:"WPI_DashboardUpdate Command Params.vi"("Update"=w232, "NewVal"=w233, "Commands"=w231, "Param Tbl"=w230) -> ()  [unwired: 7 in, 1 out]
          }
        }
        n131 = call <vilib>:"Connextion Info.vi"() -> ("Connected"=→"NT Connection":bool)  [unwired: 10 in, 1 out]
      }
      event "Set": Value Change {
        n132 = event-data() -> ()  [unwired: 1 in, 6 out]
        n133 = Boolean Array To Number(Boolean array="Array") -> (number=w254:u32)
        n134 = Number To Fractional String(number="Elbow Angle") -> (F-format string=w251:string)  [unwired: 3 in]
        n135 = Number To Fractional String(number="Wrist Angle") -> (F-format string=w249:string)  [unwired: 3 in]
        n136 = Number To Fractional String(number="Shoulder Angle") -> (F-format string=w247:string)  [unwired: 3 in]
        n137 = Number To Fractional String(number="Turret Angle") -> (F-format string=w245:string)  [unwired: 3 in]
        n138 = Number To Fractional String(number=w254) -> (F-format string=w253:string)  [unwired: 3 in]
        n139 = property on="Arm Positions" class="Enum (strict)"() -> ("Strings []"=w259:string[])  [unwired: 2 in, 2 out]
        n140 = Index Array(array=w259, index="Arm Positions") -> (element=w257:string)
        n141 = Concatenate Strings(w257, ":0," ("string"), w247, w245, w249, w251, w253) -> (w243:string)
        n142 = call <vilib>:"NT Write String.vi"("String"=w243, "Name"="Position") -> ()  [unwired: 9 in, 1 out]
      }
      event "Test Tree": Value Change {
        # "Show appropriate\ncontrols"
        n143 = event-data() -> ("CtlRef"=w265:refnum<vi>, "NewVal"=w263:string)  [unwired: 1 in]
        n144 = call <vilib>:"WPI_UtilitiesGetTreeIOName.vi"("NewVal"=w263, "TreeControl in"=w265) -> ("I/O Name"=w266:string)  [unwired: 9 in]
        n145 = case shown="\"Camera\"" w266 {
          selector: w266 -> [_ w273 _ w295 w304 _]
          tunnel: w263 -> [_ _ w292 w294 _ w311]
          tunnel: cluster{string[]}[] [{["640x480", "320x240", "160x120"]}, {["Auto", "Fixed indoor", "Fixed outdoor 1", "Fixed outdoor 2", "Fixed fluorescent 1", "Fixed fluorescent 2", "Hold current"]}, {["Auto", "Flicker-free 50 Hz", "Flicker-free 60 Hz", "Hold current"]}, {["None", "Prioritize frame rate", "Prioritize image quality"]}, {["Monochrome", "Color"]}] -> [_ _ _ _ _ w310]
          frame Default {
            w268 = FALSE ("Visible")
            w267 = FALSE ("Visible")
            n146 = property on="Motor" class="Clust (strict)"("Visible"=w267) -> ()  [unwired: 2 in, 2 out]
            n147 = property on="Test Ring" class="Ring (strict)"("Visible"=w267) -> ()  [unwired: 2 in, 2 out]
            n148 = property on="Rev/Fwd" class="Clust (strict)"("Visible"=w268) -> ()  [unwired: 2 in, 2 out]
            n149 = property on="On/Off" class="Bool (strict)"("Visible"=w268) -> ()  [unwired: 2 in, 2 out]
            n150 = property on="Test Slider" class="Slide (strict)"("Visible"=w268) -> ()  [unwired: 2 in, 2 out]
          }
          frame "Analog Out", "Motor", "PWM" {
            w274 = FALSE ("Visible")
            n151 = case shown="\"Analog Out\"" w273 {
              tunnel: [1.0 ("Value") -1.0 ("Value") 0.0 ("Value")] -> w272
              tunnel: [255.0 ("Value") 1.0 ("Value") 5.0 ("Value")] -> w271
              tunnel: [128.0 ("Value") 0.0 ("Value") 0.0 ("Value")] -> w270
              tunnel: [64.0 ("Value") 0.5 ("Value") 1.0 ("Value")] -> w269
              frame "PWM" {
              }
              frame "Motor", Default {
              }
              frame "Analog Out" {
              }
            }
            n152 = property on="Motor" class="Clust (strict)"("Visible"=TRUE) -> ()  [unwired: 2 in, 2 out]
            n153 = property on="Value" class="Slide (strict)"("Value"=w270, "Scale.Minimum"=w272, "Scale.Maximum"=w271, "Scale.Increment"=w269) -> ()  [unwired: 2 in, 2 out]
            n154 = property on="On/Off" class="Bool (strict)"("Visible"=w274) -> ()  [unwired: 2 in, 2 out]
            n155 = property on="Test Slider" class="Slide (strict)"("Visible"=w274) -> ()  [unwired: 2 in, 2 out]
            n156 = property on="Test Ring" class="Ring (strict)"("Visible"=w274) -> ()  [unwired: 2 in, 2 out]
            n157 = property on="Rev/Fwd" class="Clust (strict)"("Visible"=w274) -> ()  [unwired: 2 in, 2 out]
          }
          frame "Servo" {
            w290 = FALSE ("Visible")
            n158 = call <vilib>:"NT Read Number.vi"("Name"=w292) -> ("Numeric"=w291:dbl)  [unwired: 9 in, 1 out]
            n159 = property on="Test Slider" class="Slide (strict)"("Visible"=TRUE, "Scale.Maximum"=170.0 ("Scale.Range:Maximum")) -> ()  [unwired: 2 in, 2 out]
            n160 = local write "Test Slider"(w291) -> ()
            n161 = property on="Motor" class="Clust (strict)"("Visible"=w290) -> ()  [unwired: 2 in, 2 out]
            n162 = property on="Rev/Fwd" class="Clust (strict)"("Visible"=w290) -> ()  [unwired: 2 in, 2 out]
            n163 = property on="On/Off" class="Bool (strict)"("Visible"=w290) -> ()  [unwired: 2 in, 2 out]
            n164 = property on="Test Ring" class="Ring (strict)"("Visible"=w290) -> ()  [unwired: 2 in, 2 out]
          }
          frame "Relay", "Solenoid" {
            w293 = FALSE ("Visible")
            n165 = property on="Motor" class="Clust (strict)"("Visible"=w293) -> ()  [unwired: 2 in, 2 out]
            n166 = property on="Test Slider" class="Slide (strict)"("Visible"=w293) -> ()  [unwired: 2 in, 2 out]
            n167 = Search and Replace String(input string=w294, search string="/Value  **", replace string="/Direction") -> (result string=w300:string)  [unwired: 5 in, 3 out]
            n168 = property on="Test Ring" class="Ring (strict)"("Visible"=w293) -> ()  [unwired: 2 in, 2 out]
            n169 = call <vilib>:"NT Read String.vi"("Name"=w300) -> ("String"=w298:string)  [unwired: 9 in, 1 out]
            n170 = Equal?(x="Both directions", y=w298) -> (x = y?=w296:bool)
            n171 = Not(x=w296) -> (.not. x?=w297:bool)
            n172 = property on="Rev/Fwd" class="Clust (strict)"("Visible"=w296) -> ()  [unwired: 2 in, 2 out]
            n173 = property on="On/Off" class="Bool (strict)"("Visible"=w297, "Caption.Text"=w295) -> ()  [unwired: 2 in, 2 out]
          }
          frame "Compressor", "Digital Out" {
            w303 = FALSE ("Visible")
            # "Get direction and finish"
            n174 = property on="Motor" class="Clust (strict)"("Visible"=w303) -> ()  [unwired: 2 in, 2 out]
            n175 = property on="Test Slider" class="Slide (strict)"("Visible"=w303) -> ()  [unwired: 2 in, 2 out]
            n176 = property on="Test Ring" class="Ring (strict)"("Visible"=w303) -> ()  [unwired: 2 in, 2 out]
            n177 = property on="On/Off" class="Bool (strict)"("Visible"=TRUE, "Caption.Text"=w304) -> ()  [unwired: 2 in, 2 out]
            n178 = property on="Rev/Fwd" class="Clust (strict)"("Visible"=FALSE) -> ()  [unwired: 2 in, 2 out]
          }
          frame "Camera" {
            n179 = call <vilib>:"Get Last Path Segment.vi"("String in"=w311) -> ("String out"=w312:string)  [unwired: 10 in]
            n180 = property on="On/Off" class="Bool (strict)"("Visible"=FALSE) -> ()  [unwired: 2 in, 2 out]
            n181 = property on="Motor" class="Clust (strict)"("Visible"=FALSE) -> ()  [unwired: 2 in, 2 out]
            n182 = property on="Rev/Fwd" class="Clust (strict)"("Visible"=FALSE) -> ()  [unwired: 2 in, 2 out]
            n183 = case shown="\"White Balance  **\"" w312 {
              tunnel: w311 -> [w318 w327 w336 w345 w354 _ w360]
              tunnel: w310 -> [w316 w324 w333 w342 w351 _ _]
              frame "Size  **" {
                n184 = Index Array(array=w316) -> (element=w315:cluster{string[]})  [unwired: 1 in]
                n185 = call <vilib>:"NT Read String.vi"("Name"=w318) -> ("String"=w317:string)  [unwired: 9 in, 1 out]
                n186 = Unbundle(w315) -> (w313:string[])
                n187 = Match First String(2:w313, 3:w317) -> (0:w314:i32)  [unwired: 1 out]
                n188 = property on="Test Ring" class="Ring (strict)"("Value"=w314, "Strings []"=w313) -> ()  [unwired: 2 in, 2 out]
                n189 = property on="Test Ring" class="Ring (strict)"("Visible"=TRUE) -> ()  [unwired: 2 in, 2 out]
                n190 = property on="Test Slider" class="Slide (strict)"("Visible"=FALSE) -> ()  [unwired: 2 in, 2 out]
              }
              frame "White Balance  **" {
                n191 = Index Array(array=w324, index=1) -> (element=w325:cluster{string[]})
                n192 = call <vilib>:"NT Read String.vi"("Name"=w327) -> ("String"=w326:string)  [unwired: 9 in, 1 out]
                n193 = Unbundle(w325) -> (w322:string[])
                n194 = Match First String(2:w322, 3:w326) -> (0:w321:i32)  [unwired: 1 out]
                n195 = property on="Test Ring" class="Ring (strict)"("Value"=w321, "Strings []"=w322) -> ()  [unwired: 2 in, 2 out]
                n196 = property on="Test Ring" class="Ring (strict)"("Visible"=TRUE) -> ()  [unwired: 2 in, 2 out]
                n197 = property on="Test Slider" class="Slide (strict)"("Visible"=FALSE) -> ()  [unwired: 2 in, 2 out]
              }
              frame "Exposure  **" {
                n198 = Index Array(array=w333, index=2) -> (element=w334:cluster{string[]})
                n199 = call <vilib>:"NT Read String.vi"("Name"=w336) -> ("String"=w335:string)  [unwired: 9 in, 1 out]
                n200 = Unbundle(w334) -> (w330:string[])
                n201 = Match First String(2:w330, 3:w335) -> (0:w331:i32)  [unwired: 1 out]
                n202 = property on="Test Ring" class="Ring (strict)"("Value"=w331, "Strings []"=w330) -> ()  [unwired: 2 in, 2 out]
                n203 = property on="Test Ring" class="Ring (strict)"("Visible"=TRUE) -> ()  [unwired: 2 in, 2 out]
                n204 = property on="Test Slider" class="Slide (strict)"("Visible"=FALSE) -> ()  [unwired: 2 in, 2 out]
              }
              frame "Exposure Priority  **" {
                n205 = Index Array(array=w342, index=3) -> (element=w343:cluster{string[]})
                n206 = call <vilib>:"NT Read String.vi"("Name"=w345) -> ("String"=w344:string)  [unwired: 9 in, 1 out]
                n207 = Unbundle(w343) -> (w339:string[])
                n208 = Match First String(2:w339, 3:w344) -> (0:w340:i32)  [unwired: 1 out]
                n209 = property on="Test Ring" class="Ring (strict)"("Value"=w340, "Strings []"=w339) -> ()  [unwired: 2 in, 2 out]
                n210 = property on="Test Ring" class="Ring (strict)"("Visible"=TRUE) -> ()  [unwired: 2 in, 2 out]
                n211 = property on="Test Slider" class="Slide (strict)"("Visible"=FALSE) -> ()  [unwired: 2 in, 2 out]
              }
              frame "Color Enable  **" {
                n212 = Index Array(array=w351, index=4) -> (element=w352:cluster{string[]})
                n213 = call <vilib>:"NT Read String.vi"("Name"=w354) -> ("String"=w353:string)  [unwired: 9 in, 1 out]
                n214 = Unbundle(w352) -> (w348:string[])
                n215 = Match First String(2:w348, 3:w353) -> (0:w349:i32)  [unwired: 1 out]
                n216 = property on="Test Ring" class="Ring (strict)"("Value"=w349, "Strings []"=w348) -> ()  [unwired: 2 in, 2 out]
                n217 = property on="Test Ring" class="Ring (strict)"("Visible"=TRUE) -> ()  [unwired: 2 in, 2 out]
                n218 = property on="Test Slider" class="Slide (strict)"("Visible"=FALSE) -> ()  [unwired: 2 in, 2 out]
              }
              frame Default {
                n219 = property on="Test Ring" class="Ring (strict)"("Visible"=FALSE) -> ()  [unwired: 2 in, 2 out]
                n220 = property on="Test Slider" class="Slide (strict)"("Visible"=FALSE) -> ()  [unwired: 2 in, 2 out]
              }
              frame "Brightness  **", "Color Level  **", "Compression  **", "FPS  **", "Sharpness  **" {
                n221 = call <vilib>:"NT Read Number.vi"("Name"=w360) -> ("Numeric"=w359:dbl)  [unwired: 9 in, 1 out]
                n222 = local write "Test Slider"(w359) -> ()
                n223 = property on="Test Slider" class="Slide (strict)"("Visible"=TRUE, "Scale.Maximum"=100.0 ("Scale.Range:Maximum")) -> ()  [unwired: 2 in, 2 out]
                n224 = property on="Test Ring" class="Ring (strict)"("Visible"=FALSE) -> ()  [unwired: 2 in, 2 out]
              }
            }
          }
        }
        n225 = property on="Progress" class="Clust (strict)"("Visible"=FALSE) -> ()  [unwired: 2 in, 2 out]
      }
      event "Test Name": Mouse Enter {
        # "Populate the ring with the list of tests"
        n226 = event-data() -> ()  [unwired: 1 in, 1 out]
        n227 = call <vilib>:"NT Read String Array.vi"("Name"="TestMode/TestList") -> ("String Array"=w368:string[])  [unwired: 9 in, 1 out]
        n228 = Build Array (concatenate)("Select the test to run...", w368) -> (w367:string[])
        n229 = property on="Test Name" class="Ring (strict)"("Strings []"=w367) -> ()  [unwired: 2 in, 2 out]
      }
      event "Test Name": Value Change {
        w370 = FALSE ("Visible")
        # "Tell the robot the test name to run"
        n230 = event-data() -> ("NewVal"=w374:u16)  [unwired: 1 in]
        n231 = property on="Test Name" class="Ring (strict)"() -> ("Strings []"=w375:string[])  [unwired: 2 in, 2 out]
        n232 = local write "Progress"(T7 {"Test Progress"=0, "Test Progress Text"=""} ("Progress")) -> ()
        n233 = Index Array(array=w375, index=w374) -> (element=w373:string)
        n234 = call <vilib>:"NT Write String.vi"("String"=w373, "Name"="TestMode/TestName") -> ()  [unwired: 9 in, 1 out]
        n235 = property on="Progress" class="Clust (strict)"("Visible"=TRUE) -> ()  [unwired: 2 in, 2 out]
        n236 = property on="Motor" class="Clust (strict)"("Visible"=w370) -> ()  [unwired: 2 in, 2 out]
        n237 = property on="Test Slider" class="Slide (strict)"("Visible"=w370) -> ()  [unwired: 2 in, 2 out]
        n238 = property on="On/Off" class="Bool (strict)"("Visible"=w370) -> ()  [unwired: 2 in, 2 out]
        n239 = property on="Rev/Fwd" class="Clust (strict)"("Visible"=w370) -> ()  [unwired: 2 in, 2 out]
        n240 = property on="Test Ring" class="Ring (strict)"("Visible"=w370) -> ()  [unwired: 2 in, 2 out]
      }
      event "Select Auto": Mouse Enter {
        # "Populate the combo box with the list of autonomous options"
        n241 = event-data() -> ()  [unwired: 1 in, 1 out]
        n242 = call <vilib>:"NT Read String Array.vi"("Name"="Auto List") -> ("String Array"=w377:string[])  [unwired: 9 in, 1 out]
        n243 = property on="Select Auto" class="CmbBox"("Strings[]"=w377) -> ()  [unwired: 2 in, 2 out]
      }
      event "Select Auto": Value Change {
        # "User modified the Auto Selection. Write to NT variable so robot knows."
        n244 = event-data() -> ("NewVal"=w380:string)  [unwired: 1 in]
        n245 = call <vilib>:"NT Write String.vi"("String"=w380, "Name"="Auto Selector") -> ()  [unwired: 9 in, 1 out]
      }
      event "Command Selection": Value Change {
        # "Get the params and show in table"
        n246 = event-data() -> ("NewVal"=w386:i32)  [unwired: 1 in]
        n247 = property on="Command Selection" class="MCListbox (strict)"() -> ("ItemNames"=w384:string[][])  [unwired: 2 in, 2 out]
        n248 = call <vilib>:"WPI_DashboardUpdate Command Params.vi"("NewVal"=w386, "Commands"=w384, "Param Tbl"=w385) -> ()  [unwired: 8 in, 1 out]
      }
      event "Execute Command": Value Change {
        # "Started one, Unique ID holds\nresponse"
        n249 = event-data() -> ()  [unwired: 1 in, 1 out]
        n250 = property on="Command Selection" class="MCListbox (strict)"() -> ("ItemNames"=w397:string[][])  [unwired: 2 in, 2 out]
        n251 = Index Array(array=w397, index (row)="Command Selection", index (col)=0) -> (element=w395:string)
        n252 = call <vilib>:"Invoke Commands.vi"("Command Params"="Command Params", "Function Name"=w395) -> ("Params"=w391:u8, "Started"=w390:bool)  [unwired: 7 in, 1 out]
        n253 = Array Subset(array="Command Params", length (row)=w391) -> (w392:string[][])  [unwired: 3 in]
        n254 = Select(t="Executing" ("Cmd Status"), s=w390, f="" ("Cmd Status")) -> (s? t:f=→"Cmd Status":string)
      }
      event "Command Selection": Double Click {
        n255 = event-data() -> ("Row"=w405:i32)  [unwired: 1 in]
        n256 = property on="Command Selection" class="MCListbox (strict)"() -> ("ItemNames"=w408:string[][])  [unwired: 2 in, 2 out]
        n257 = local read "Command Params"() -> (w404:string[][])
        n258 = Index Array(array=w408, index (row)=w405, index (col)=0) -> (element=w406:string)
        n259 = call <vilib>:"Invoke Commands.vi"("Command Params"=w404, "Function Name"=w406) -> ("Params"=w403:u8, "Started"=w398:bool)  [unwired: 7 in, 1 out]
        n260 = Array Subset(array=w404, length (row)=w403) -> (w402:string[][])  [unwired: 3 in]
        n261 = Select(t="Executing" ("Cmd Status"), s=w398, f="" ("Cmd Status")) -> (s? t:f=w399:string)
        n262 = local write "Cmd Status"(w399) -> ()
      }
      event "CheckList": Double Click {
        # "Shift clears all"
        # "Update symbols on the listbox"
        n263 = event-data() -> ("PlatMods.Shift"=w410:bool, "Row"=w412:i32)  [unwired: 1 in]
        n264 = case shown="True" w410 {
          tunnel: w412 -> [w416 _]
          tunnel: 1 -> [w415 _]
          frame False {
            n265 = property on="CheckList" class="LstBox (strict)"() -> ("Item Symbols"=w414:i32[])  [unwired: 2 in, 2 out]
            n266 = Replace Array Subset(array=w414, new element=w415, index=w416) -> (w413:i32[])
            n267 = property on="CheckList" class="LstBox (strict)"("Item Symbols"=w413) -> ()  [unwired: 2 in, 2 out]
          }
          frame True {
            w417 = 0 ("Top Row")
            n268 = property on="CheckList" class="LstBox (strict)"() -> ("Number of Rows"=w419:u32)  [unwired: 2 in, 2 out]
            n269 = Initialize Array(0, w419) -> (w418:i32[])
            n270 = property on="CheckList" class="LstBox (strict)"("Top Row"=w417, "Value"=w417, "Item Symbols"=w418) -> ()  [unwired: 2 in, 2 out]
          }
        }
      }
      event "CheckList": Key Down {
        # "Update symbols on the listbox\nLeft and right keys check and uncheck"
        n271 = event-data() -> ("VKey"=w423:T23)  [unwired: 1 in]
        n272 = case shown="\"Left\", \"Right\"" w423 {
          selector: w423 -> [w428 _]
          tunnel: eventvkey."Left" ("VKey") -> [w426 _]
          frame "Left", "Right" {
            n273 = Equal?(x=w426, y=w428) -> (x = y?=w427:bool)
            n274 = Select(t=0, s=w427, f=1) -> (s? t:f=w429:i32)
            n275 = property on="CheckList" class="LstBox (strict)"() -> ("Item Symbols"=w432:i32[])  [unwired: 2 in, 2 out]
            n276 = Replace Array Subset(array=w432, new element=w429, index="CheckList") -> (w431:i32[])
            n277 = property on="CheckList" class="LstBox (strict)"("Item Symbols"=w431) -> ()  [unwired: 2 in, 2 out]
          }
          frame Default {
          }
        }
      }
      event "Motor.Enable": Value Change {
        # "When the test mode otor enable helper is set, update that\ntree row item's value"
        n278 = event-data() -> ("NewVal"=w438:bool)  [unwired: 1 in]
        n279 = Unbundle("Motor") -> ("Value"=w437:dbl)  [unwired: 1 out]
        n280 = Select(t=w437, s=w438, f=0.0) -> (s? t:f=w435:dbl)
        n281 = call <vilib>:"NT Write Number.vi"("Numeric"=w435, "Name"=w434) -> ()  [unwired: 9 in, 1 out]
      }
      event "Test Slider": Value Change {
        # "When the test mode slider helper is set, update that\ntree row item's value"
        n282 = event-data() -> ("NewVal"=w441:dbl)  [unwired: 1 in]
        n283 = call <vilib>:"NT Write Number.vi"("Numeric"=w441, "Name"=w442) -> ()  [unwired: 9 in, 1 out]
      }
      event "On/Off": Value Change {
        # "When the test mode on/off helper value is set, update that\ntree row item's value"
        n284 = event-data() -> ("NewVal"=w446:bool)  [unwired: 1 in]
        n285 = Boolean To (0,1)(Boolean=w446) -> (0, 1=w445:i16)
        n286 = call <vilib>:"NT Write Number.vi"("Numeric"=w445, "Name"=w444) -> ()  [unwired: 9 in, 1 out]
      }
      event "Rev/Fwd": Value Change {
        # "When the test mode helper value for relays is set, update that\ntree row item's value"
        n287 = event-data() -> ("NewVal.Forward"=w454:bool, "NewVal.Reverse"=w453:bool)  [unwired: 1 in]
        n288 = Boolean To (0,1)(Boolean=w454) -> (0, 1=w450:i16)
        n289 = Boolean To (0,1)(Boolean=w453) -> (0, 1=w452:i16)
        n290 = Negate(x=w452) -> (-x=w451:i16)
        n291 = Add(x=w450, y=w451) -> (x+y=w449:i16)
        n292 = call <vilib>:"NT Write Number.vi"("Numeric"=w449, "Name"=w448) -> ()  [unwired: 9 in, 1 out]
      }
      event "Test Ring": Value Change {
        # "When a test mode helper value is selected from the ring,\nset the tree item's variable to the string value"
        n293 = event-data() -> ("NewVal"=w458:u16)  [unwired: 1 in]
        n294 = property on="Test Ring" class="Ring (strict)"() -> ("Strings []"=w459:string[])  [unwired: 2 in, 2 out]
        n295 = Index Array(array=w459, index=w458) -> (element=w457:string)
        n296 = call <vilib>:"NT Write String.vi"("String"=w457, "Name"=w456) -> ()  [unwired: 9 in, 1 out]
      }
      event "Rec Mode": Value Change {
        # "Update globals for recording mode and path to read log from.\nClear when logging and let NetworkTables set path for vision to\nuse."
        n297 = event-data() -> ("NewVal"=w470:enum32{"Stop", "Record", "Playback"})  [unwired: 1 in]
        n298 = global write "WPI_DashboardLogging Global.vi" "Logging Filename"(path "") -> ()
        n299 = global write "WPI_DashboardLogging Global.vi" "Recording"(w470) -> ()
        n300 = case shown="\"Playback\"" w470 {
          tunnel: w469 -> [_ w472 w481]
          tunnel: [_ _ w480] -> w467
          tunnel: [_ _ w479] -> _
          tunnel: w465 -> [_ _ w477]
          tunnel: cluster{i32, i32} {-250, 170} -> [_ _ w476]
          tunnel: [_ _ T24 {"Image Size"=TRUE, "Image Type"=TRUE, "Pixel Value"=TRUE, "ROI Information"=TRUE, "Zoom Factor"=FALSE} ("Image Information Shown:All Elements")] -> w460
          tunnel: [_ _ TRUE ("Zoom Factor")] -> w461
          tunnel: w463 -> [_ _ w473]
          frame Default {
          }
          frame "Stop", "Record" {
            # "Place Window too"
            n301 = invoke class="VI" method="FP.Close"(reference=w472) -> (reference out=w471:refnum<vi>)  [unwired: 2 in, 2 out]
            n302 = invoke class="VI" method="Abort VI"(reference=w471) -> ()  [unwired: 2 in, 3 out]
          }
          frame "Playback" {
            n303 = call "Open Playback Panel.vi"("Offset"=w476, "DB VI Ref"=w477, "Playback in"=w481) -> ("Playback out"=w478:refnum<vi>)  [unwired: 8 in]
            n304 = register-events(w478, w473) -> (reference out=w480:refnum<event-registration>, error out=w479:errorcluster)  [unwired: 2 in]
          }
        }
        n305 = property on="Camera Image Right" class="ImageControl"("Image Information Shown"=w460, "Image Information Visible"=w461) -> ()  [unwired: 2 in, 2 out]
        n306 = property on="Camera Image" class="ImageControl"("Image Information Shown"=w460, "Image Information Visible"=w461) -> ()  [unwired: 2 in, 2 out]
        n307 = call <vilib>:"WPI_DashboardNT Log FieldName Cache.vi"("Operation"=enum16{"Lookup/Add", "Index", "Clear"}."Clear") -> ()  [unwired: 8 in, 3 out]
      }
      event Panel Close {
        w483 = enum32{"Stop", "Record", "Playback"}."Stop" ("Rec Mode")
        # "Playback window has been closed, abort"
        n308 = event-data() -> ()  [unwired: 1 in, 4 out]
        n309 = local write "Rec Mode"(w483) -> ()
        n310 = global write "WPI_DashboardLogging Global.vi" "Recording"(w483) -> ()
      }
      event Panel Close {
        # "Abort playback window and ourself"
        n311 = event-data() -> ()  [unwired: 1 in, 4 out]
        n312 = invoke class="VI" method="FP.Close"(reference=w487) -> (reference out=w486:refnum<vi>)  [unwired: 2 in, 2 out]
        n313 = invoke class="VI" method="Abort VI"(reference=w486) -> (error out=w485:errorcluster)  [unwired: 2 in, 2 out]
        n314 = invoke class="VI" method="Abort VI"(error in=w485) -> ()  [unwired: 2 in, 3 out]
      }
      event User Event {
        n315 = event-data() -> ("IDs"=w494:cluster{"RPC field ID":u16, "Unique ID":u16}, "String"=w493:string)  [unwired: 1 in]
        n316 = Bundle("IDs"=w494, "String"=w493) -> (w492:T10)  [unwired: 1 in]
        n317 = call <vilib>:"Retrieve RPC Response.vi"("RPC Response"=w492) -> ("Output"=w490:string[][])  [unwired: 10 in]
        n318 = Build Array (concatenate)(w488, w490) -> (w489:string[][])
        n319 = local write "Command Params"(w489) -> ()
        n320 = local write "Cmd Status"("" ("Cmd Status")) -> ()
      }
      event "Tree": Double Click {
        n321 = event-data() -> ("PlatMods"=w500:T27, "Tag"=w497:string)  [unwired: 1 in]
        n322 = Unbundle(w500) -> ("Shift"=w499:bool)  [unwired: 4 out]
        n323 = String Subset(string=w497, length (rest)=1 ("length (rest)")) -> (substring=w496:string)  [unwired: 1 in]
        n324 = Not(x=w499) -> (.not. x?=w498:bool)
        n325 = case shown="\"/\"" w496 {
          tunnel: w497 -> [_ w503]
          tunnel: w498 -> [_ w502]
          frame Default {
          }
          frame "/" {
            n326 = call <vilib>:"NT Update Persistence.vi"("Persistence"=w502, "Name"=w503) -> ()  [unwired: 9 in, 1 out]
          }
        }
      }
    }
  }
  n327 = while {
    tunnel: w65 -> [w505]
    i -> [w508]
    stop <- FALSE stop-if-true
    n328 = Wait (ms)(milliseconds to wait=u32 100) -> ()  [unwired: 1 out]
    n329 = case shown="\"Playback\"" "Rec Mode" {
      tunnel: w508 -> [_ _ w523]
      tunnel: [u32 2829099 ("Base Color") u32 11141120 ("Target Color") w512] -> w504
      frame "Stop", Default {
        # "Reset the color, extra updates don't cost much"
      }
      frame "Record" {
      }
      frame "Playback" {
        # "Playback"
        n330 = Quotient & Remainder(x=w523, y=u32 50 ("milliseconds to wait")) -> (x-y*floor(x/y)=w519:u32)  [unwired: 1 out]
        n331 = Divide(x=w519, y=u32 50 ("milliseconds to wait")) -> (x/y=w516:dbl)
        n332 = Multiply(x=6.283185307179586, y=w516) -> (x*y=w521:dbl)
        n333 = Sine(x=w521) -> (sin(x)=w520:dbl)
        n334 = Absolute Value(x=w520) -> (abs(x)=w513:dbl)
        n335 = call "Interpolate RGB Color.vi"("Proportion"=w513, "Target Color"=u32 30976, "Base Color"=u32 2829099) -> ("Result Color"=w512:u32)  [unwired: 8 in]
      }
    }
    n336 = property class="Pane"(reference=w505, "PaneColor"=w504) -> ()  [unwired: 1 in, 2 out]
  }
  n337 = local write "Dashboard Tab"(T2."Drive" ("Dashboard Tab")) -> ()
  n338 = property on="On/Off" class="Bool (strict)"("Visible"=w36) -> ()  [unwired: 2 in, 2 out]
  n339 = property on="Motor" class="Clust (strict)"("Visible"=w36) -> ()  [unwired: 2 in, 2 out]
  n340 = property on="Progress" class="Clust (strict)"("Visible"=w36) -> ()  [unwired: 2 in, 2 out]
  n341 = property on="Test Ring" class="Ring (strict)"("Visible"=w36) -> ()  [unwired: 2 in, 2 out]
  n342 = property on="Rev/Fwd" class="Clust (strict)"("Visible"=w36) -> ()  [unwired: 2 in, 2 out]
  n343 = while {
    tunnel: u16 1741 ("timeout ms (25000)") -> [w525]
    stop <- FALSE stop-if-true
    n344 = TCP Create Listener(10:w525) -> (0:w524:errorcluster, 3:w526:refnum<k5>)  [unwired: 4 in, 1 out]
    n345 = case shown="No Error" w524 {
      selector: w524 -> [w528 _]
      tunnel: w526 -> [w529 _]
      frame No Error {
        n346 = while {
          tunnel: w529 -> [w532]
          tunnel: w528 -> [w531]
          stop <- FALSE stop-if-true
          n347 = TCP Wait On Listener(8:w531, 11:w532) -> (0:w533:errorcluster, 4:w534:refnum<k5>)  [unwired: 2 in, 3 out]
          n348 = local write "TCP"(w534) -> ()
          n349 = case shown="No Error" w533 {
            frame No Error {
            }
            frame Error {
              n350 = Wait (ms)(milliseconds to wait=u32 1000) -> ()  [unwired: 1 out]
            }
          }
        }
      }
      frame Error {
        n351 = Wait (ms)(milliseconds to wait=u32 1000) -> ()  [unwired: 1 out]
      }
    }
  }
  n352 = local write "Command Selection"(u16 0 ("milliseconds to wait")) -> ()
  n353 = local write "Command Params"(string[][] [] ("Command Params")) -> ()
  n354 = global write "WPI_DashboardLogging Global.vi" "Recording"(w59) -> ()
  n355 = local write "Rec Mode"(w59) -> ()
  n356 = call <vilib>:"NT Write String.vi"("String"="Select Auto", "Name"="Auto Selector") -> ()  [unwired: 9 in, 1 out]
